vi "Usermgt.vi"(8 "error In":errorcluster) -> (0 "error out":errorcluster)   [LabVIEW 2015]
uses:
  Um- Save.ctl
  Um-Delete.ctl
  Um-Exit.ctl
  <vilib>/addons/database/Connection.llb/DB Tools Open Connec (String).vi
  <vilib>/addons/database/_DB Variant To Data/Database Variant To Data.xnode
  <vilib>/addons/database/NI_Database_API.lvlib
panel:
  in  "Operator ID":string
  out "data":string[](array[string])
  out "User Name 2":string
  out "error out 2":errorcluster
  in  "Exit":T1
  in  "Deleat":T2
  in  "Save":T3
  in  "User Type":string
  in  "User Type":u16(ring) items=["Operator", "Supervisor", "admin"]
  in  "Re-Password":string
  in  "Password":string
  in  "User Name":string
  in  "User Table":i32(listbox)
  # "User Create"
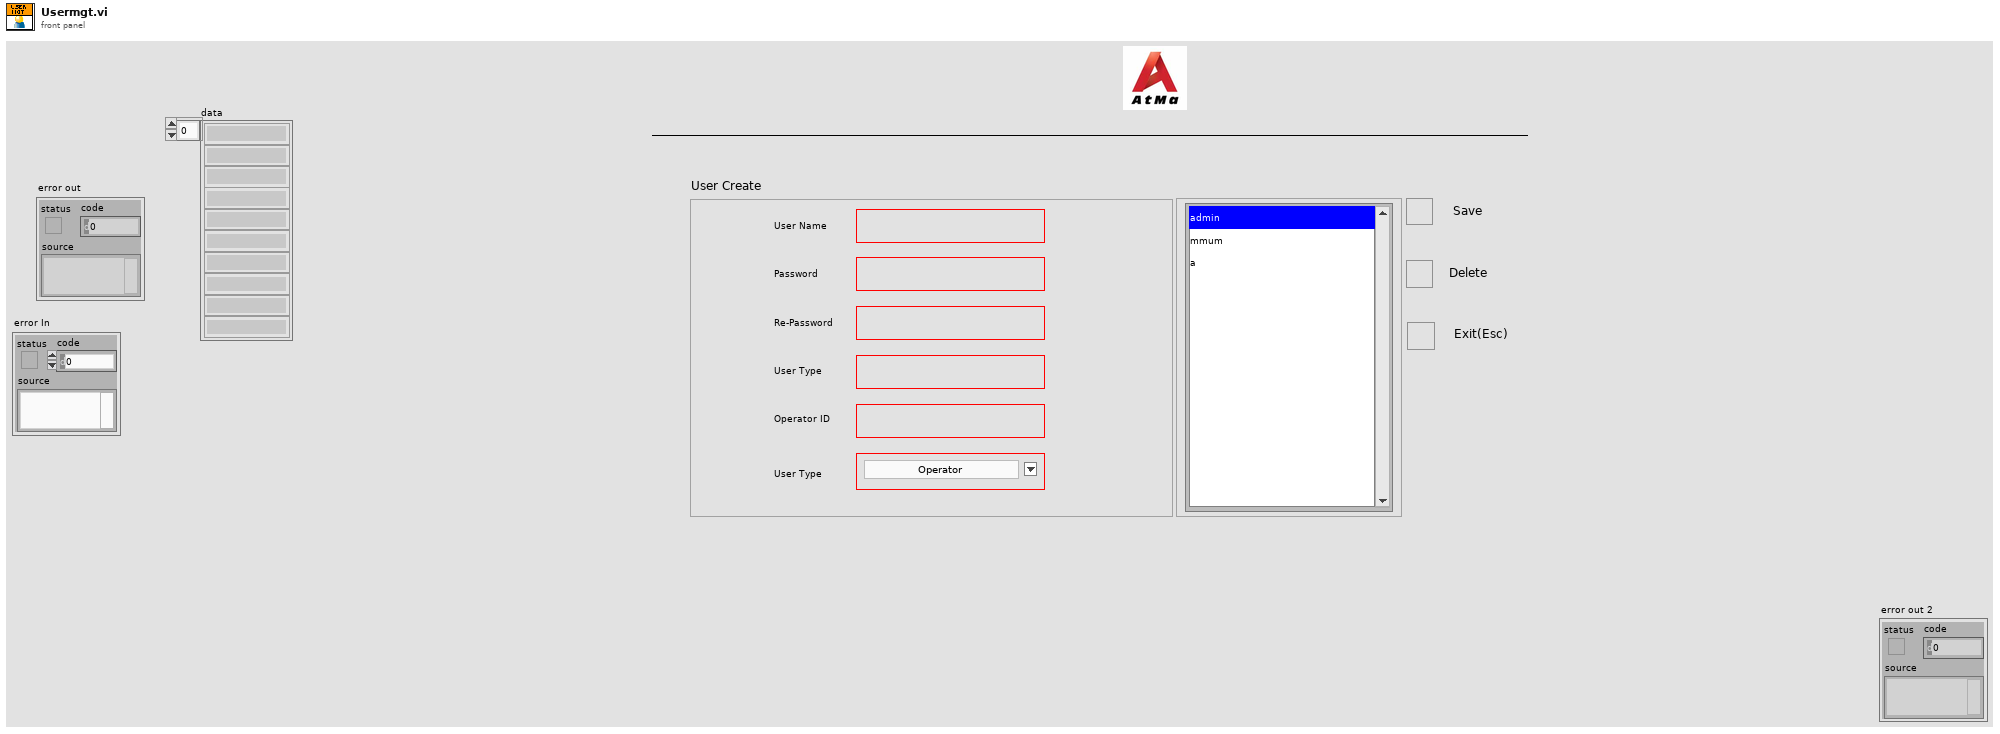
[diagram p1: front panel]
types:
  T1 = typedef "Um-Exit.ctl" = bool
  T2 = typedef "Um-Delete.ctl" = bool
  T3 = typedef "Um- Save.ctl" = bool
  T4 = cluster{"User Name":string, "Password":string, "User Type":string}
  T5 = typedef "NI_Database_API.lvlib/Conn ObjectReference.ctl" = refnum<k1>
  T6 = cluster{"User Name":string, "Password":string, "User Type":string, "Access right":string}
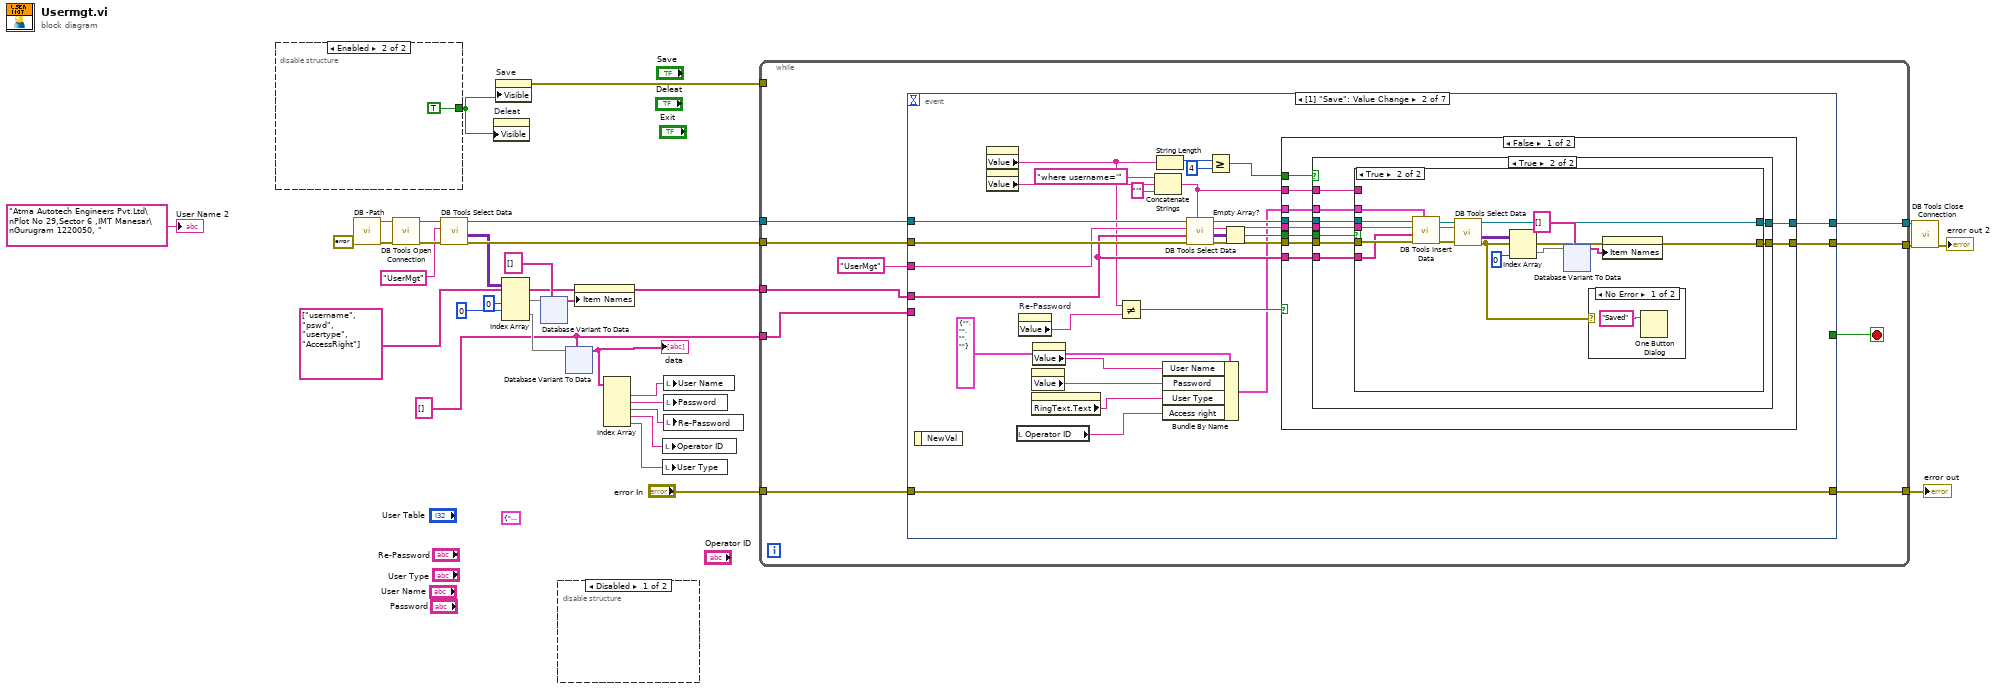
[diagram p0: block diagram]
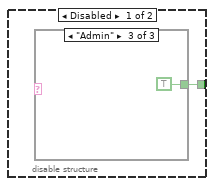
[diagram p3: hidden frame]
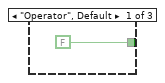
[diagram p4: hidden frame]
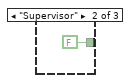
[diagram p5: hidden frame]
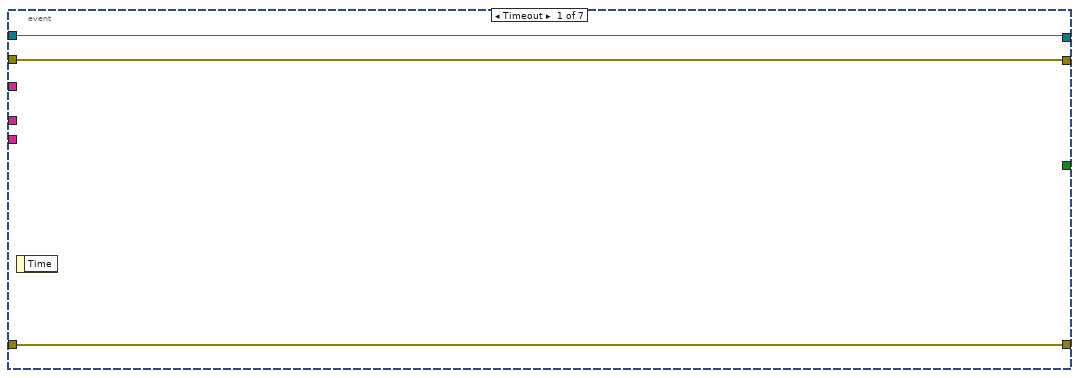
[diagram p6: hidden frame]
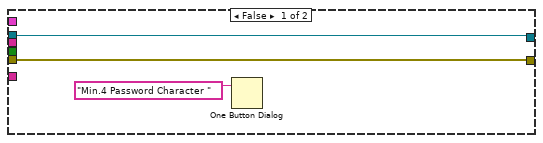
[diagram p7: hidden frame]
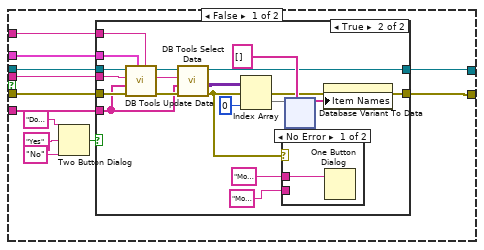
[diagram p8: hidden frame]
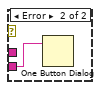
[diagram p10: hidden frame]
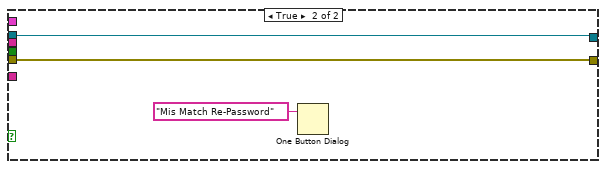
[diagram p12: hidden frame]
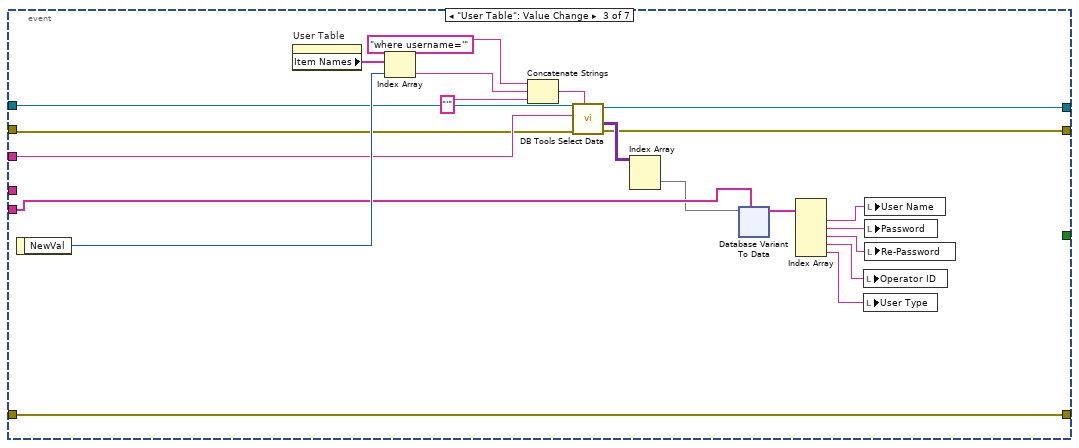
[diagram p13: hidden frame]
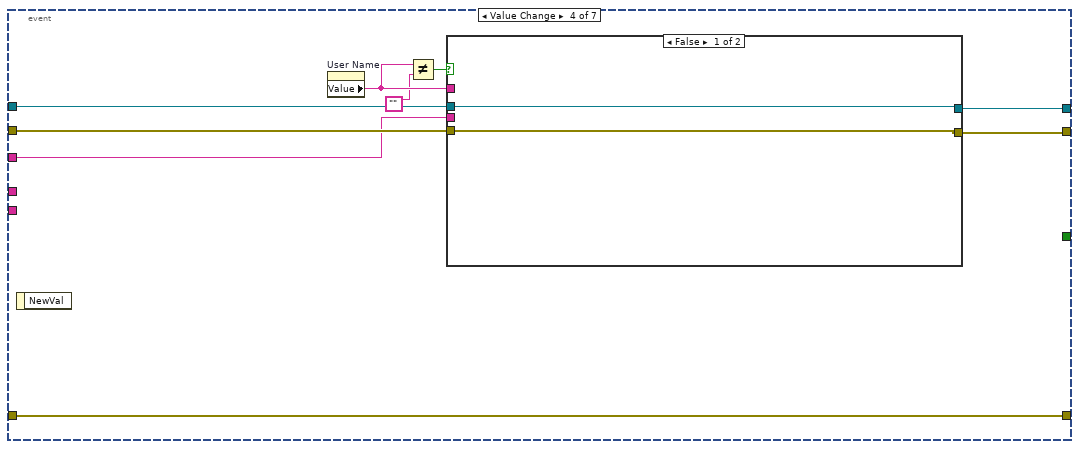
[diagram p14: hidden frame]
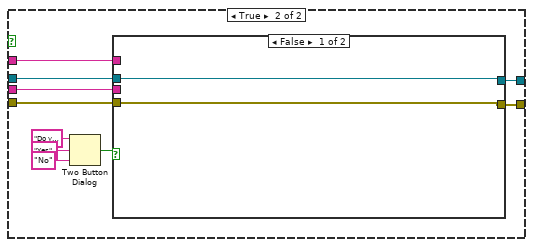
[diagram p15: hidden frame]
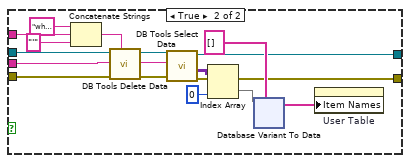
[diagram p16: hidden frame]
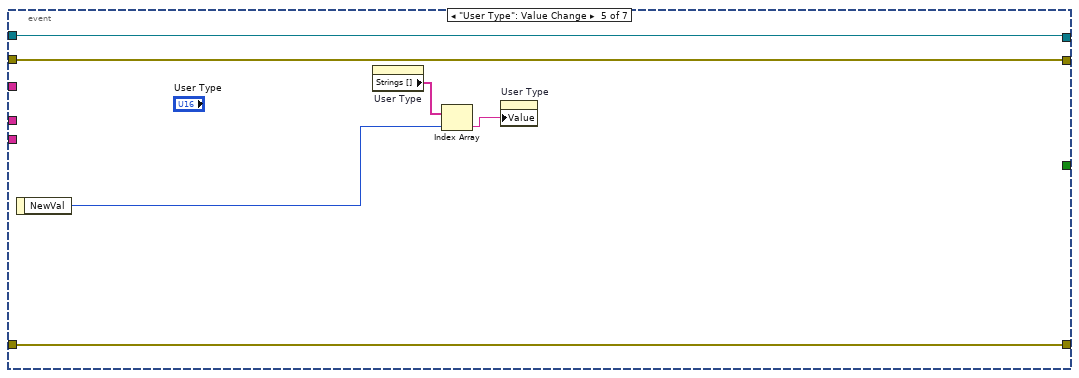
[diagram p17: hidden frame]
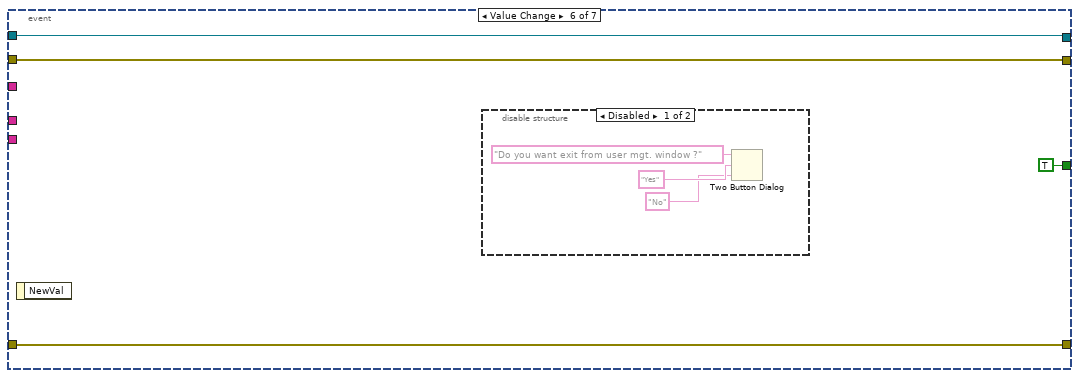
[diagram p18: hidden frame]
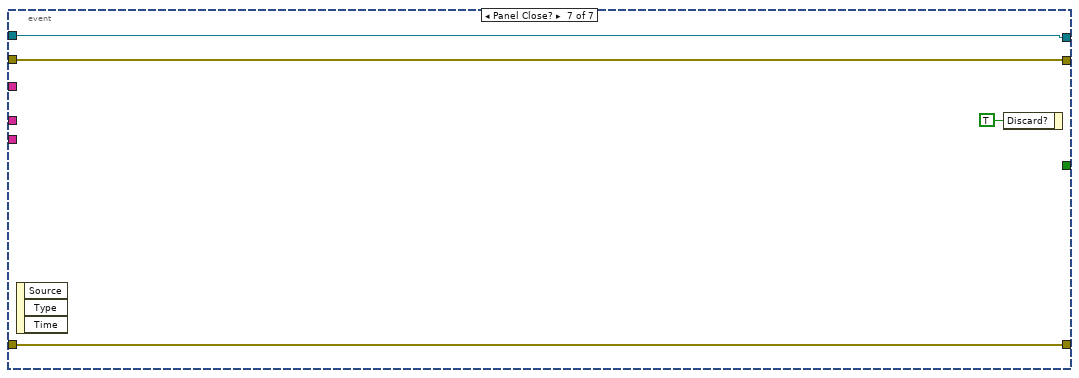
[diagram p20: hidden frame]
diagram:
  w1 = string[] [] ("columns")
  (unwired) T4 {"User Name"="", "Password"="", "User Type"=""} ("Input data")
  n1 = disable-structure shown="Enabled" {
    disable-tunnel: [w31 TRUE] -> w17
    frame Disabled {
      n2 = case shown="\"Admin\"" {
        selector: _ -> [_ _ _]
        tunnel: [FALSE FALSE TRUE] -> w31
        frame "Operator", Default {
        }
        frame "Supervisor" {
        }
        frame "Admin" {
        }
      }
    }
    frame Enabled {
    }
  }
  n3 = call "DB -Path.vi"() -> ("String"=w30:string)  [unwired: 11 in]
  n4 = call-poly <vilib>:"DB Tools Open Connection.vi"("error in (no error)"=errorcluster {"status"=FALSE, "code"=0, "source"=""}, "connection information"=w30) -> ("error out"=w27:errorcluster, "connection reference"=w26:T5)  [unwired: 6 in]
  n5 = call <vilib>:"DB Tools Select Data.vi"("error in (no error)"=w27, "table"="UserMgt", "connection reference"=w26) -> ("error out"=w24:errorcluster, "data"=w18:variant[][], "connection reference out"=w25:T5)  [unwired: 3 in]
  n6 = property on="Deleat" class="Bool (strict)"("Visible"=w17) -> ()  [unwired: 2 in, 2 out]
  n7 = property on="Save" class="Bool (strict)"("Visible"=w17) -> (error out=w16:errorcluster)  [unwired: 2 in, 1 out]
  n8 = Index Array(array=w18, index (col) #1=0 ("disabled index (col)"), index (row) #2=0 ("disabled index (row)")) -> (element #1=w22:variant[], element #2=w8:variant[])  [unwired: 2 in]
  n9 = xnode "Database Variant To Data"("database variant"=w22, "type"=string[] []) -> ("data"=w19:string[])  [unwired: 1 in, 1 out]
  n10 = disable-structure shown="Disabled" {
    frame Disabled {
    }
    frame Enabled {
    }
  }
  n11 = xnode "Database Variant To Data"("database variant"=w8, "type"=w1) -> ("data"=w7:string[])  [unwired: 1 in, 1 out]
  "data" <- w7
  n12 = property on="User Table" class="LstBox (strict)"("Item Names"=w19) -> ()  [unwired: 2 in, 2 out]
  n13 = Index Array(array=w7) -> (element #1=w6:string, element #2=w5:string, element #3=w4:string, element #4=w2:string, element #5=w3:string)  [unwired: 5 in]
  n14 = local write "Operator ID"(w2) -> ()
  n15 = local write "User Type"(w3) -> ()
  n16 = local write "User Name"(w6) -> ()
  n17 = local write "Password"(w5) -> ()
  n18 = local write "Re-Password"(w4) -> ()
  n19 = while {
    tunnel: w25 -> [w44]
    tunnel: w24 -> [w43]
    tunnel: [w41] -> w29
    tunnel: [w40] -> w28
    tunnel: w16 -> [_]
    tunnel: string[] ["username", "pswd", "usertype", "AccessRight"] ("columns") -> [w39]
    tunnel: "error In" -> [w38]
    tunnel: [w37] -> w12
    tunnel: w1 -> [w36]
    stop <- w45 stop-if-true
    n20 = event shown="[1] \"Save\": Value Change" {
      selector: _ -> [_ _ _ _ _ _ _]
      dyn-events: _ -> [_ _ _ _ _ _ _]
      timeout: _ -> [_ _ _ _ _ _ _]
      tunnel: [_ _ _ _ _ TRUE ("T button?") _] -> w45
      tunnel: w44 -> [w48 w75 w237 w292 w363 w370 w375]
      tunnel: w43 -> [w47 w74 w236 w291 w362 w369 w374]
      tunnel: "UserMgt" ("table") -> [_ w67 w239 w287 _ _ _]
      tunnel: w39 -> [_ w66 _ _ _ _ _]
      tunnel: [w48 w65 w235 w285 w363 w370 w375] -> w41
      tunnel: [w47 w64 w234 w284 w362 w369 w374] -> w40
      tunnel: w38 -> [w46 w50 w233 w286 w361 w367 w376]
      tunnel: [w46 w50 w233 w286 w361 w367 w376] -> w37
      tunnel: w36 -> [_ _ w227 _ _ _ _]
      event Timeout {
        n21 = event-data() -> ()  [unwired: 1 in, 1 out]
      }
      event Value Change {
        n22 = event-data() -> ()  [unwired: 1 in, 1 out]
        n23 = property on="Password" class="Str"() -> ("Value"=w52:string)  [unwired: 2 in, 2 out]
        n24 = property on="User Name" class="Str"() -> ("Value"=w51:string)  [unwired: 2 in, 2 out]
        n25 = local read "Operator ID"() -> (w49:string)
        n26 = property on="Re-Password" class="Str"() -> ("Value"=w58:string)  [unwired: 2 in, 2 out]
        n27 = property on="User Type" class="Ring (strict)"() -> ("RingText.Text"=w55:string)  [unwired: 2 in, 2 out]
        n28 = property on="Password" class="Str"() -> ("Value"=w57:string)  [unwired: 2 in, 2 out]
        n29 = property on="User Name" class="Str"() -> ("Value"=w56:string)  [unwired: 2 in, 2 out]
        n30 = Not Equal?(x=w52, y=w58) -> (x != y?=w59:bool)
        n31 = Concatenate Strings("where username='" ("condition"), w51, "'" ("User Name")) -> (w63:string)
        n32 = String Length(string=w52) -> (length=w62:i32)
        n33 = Bundle By Name(cluster=T6 {"User Name"="", "Password"="", "User Type"="", "Access right"=""} ("input cluster"), "User Name"=w56, "Password"=w57, "User Type"=w55, "Access right"=w49) -> (w53:T6)
        n34 = call <vilib>:"DB Tools Select Data.vi"("condition"=w63, "error in (no error)"=w74, "columns"=w66, "table"=w67, "connection reference"=w75) -> ("error out"=w68:errorcluster, "data"=w73:variant[][], "connection reference out"=w69:T5)  [unwired: 1 in]
        n35 = Greater Or Equal?(x=w62, y=4) -> (x >= y?=w60:bool)
        n36 = Empty Array?(array=w73) -> (empty?=w72:bool)
        n37 = case shown="False" w59 {
          tunnel: w72 -> [w85 _]
          tunnel: w69 -> [w84 w224]
          tunnel: w68 -> [w83 w223]
          tunnel: w67 -> [w82 _]
          tunnel: w66 -> [w81 _]
          tunnel: w53 -> [w80 _]
          tunnel: [w79 w224] -> w65
          tunnel: [w78 w223] -> w64
          tunnel: w63 -> [w77 _]
          tunnel: w60 -> [w76 _]
          frame False {
            n38 = case shown="True" w76 {
              tunnel: w85 -> [_ w97]
              tunnel: w84 -> [w88 w96]
              tunnel: w83 -> [w87 w95]
              tunnel: w82 -> [_ w94]
              tunnel: w81 -> [_ w93]
              tunnel: w80 -> [_ w92]
              tunnel: [w88 w91] -> w79
              tunnel: [w87 w90] -> w78
              tunnel: w77 -> [_ w89]
              frame False {
                n39 = One Button Dialog(message="Min.4 Password Character ") -> ()  [unwired: 1 in, 1 out]
              }
              frame True {
                n40 = case shown="True" w97 {
                  tunnel: w96 -> [w109 w182]
                  tunnel: w95 -> [w108 w181]
                  tunnel: w94 -> [w103 w176]
                  tunnel: w93 -> [w100 w180]
                  tunnel: w92 -> [w101 w179]
                  tunnel: [w99 w170] -> w91
                  tunnel: [w98 w169] -> w90
                  tunnel: w89 -> [w102 _]
                  frame False {
                    n41 = Two Button Dialog(message="Do you want  modification" ("T button name (\"OK\")"), 1:"No" ("F button name (\"Cancel\")"), 2:"Yes" ("T button name (\"OK\")")) -> (T button?=w107:bool)
                    n42 = case shown="True" w107 {
                      tunnel: w109 -> [w111 w128]
                      tunnel: w108 -> [w110 w127]
                      tunnel: w103 -> [_ w122]
                      tunnel: w102 -> [_ w126]
                      tunnel: w101 -> [_ w125]
                      tunnel: w100 -> [_ w116]
                      tunnel: [w111 w115] -> w99
                      tunnel: [w110 w114] -> w98
                      frame False {
                      }
                      frame True {
                        n43 = call <vilib>:"DB Tools Update Data.vi"("condition"=w126, "data"=w125, "error in (no error)"=w127, "columns"=w116, "table"=w122, "connection reference"=w128) -> ("error out"=w123:errorcluster, "connection reference out"=w124:T5)  [unwired: 4 in]
                        n44 = call <vilib>:"DB Tools Select Data.vi"("error in (no error)"=w123, "columns"=w116, "table"=w122, "connection reference"=w124) -> ("error out"=w114:errorcluster, "data"=w121:variant[][], "connection reference out"=w115:T5)  [unwired: 2 in]
                        n45 = Index Array(array=w121, index (col)=0 ("disabled index (col)")) -> (element=w119:variant[])  [unwired: 1 in]
                        n46 = case shown="No Error" w114 {
                          tunnel: "Modification is Successfully" ("T button name (\"OK\")") -> [w129 _]
                          tunnel: "Modification is Unsuccessfully" ("T button name (\"OK\")") -> [_ w130]
                          frame No Error {
                            n47 = One Button Dialog(message=w129) -> ()  [unwired: 1 in, 1 out]
                          }
                          frame Error {
                            n48 = One Button Dialog(message=w130) -> ()  [unwired: 1 in, 1 out]
                          }
                        }
                        n49 = xnode "Database Variant To Data"("database variant"=w119, "type"=string[] []) -> ("data"=w117:string[])  [unwired: 1 in, 1 out]
                        n50 = property on="User Table" class="LstBox (strict)"("Item Names"=w117) -> ()  [unwired: 2 in, 2 out]
                      }
                    }
                  }
                  frame True {
                    n51 = call <vilib>:"DB Tools Insert Data.vi"("data"=w179, "error in (no error)"=w181, "columns"=w180, "table"=w176, "connection reference"=w182) -> ("error out"=w177:errorcluster, "connection reference out"=w178:T5)  [unwired: 5 in]
                    n52 = call <vilib>:"DB Tools Select Data.vi"("error in (no error)"=w177, "table"=w176, "connection reference"=w178) -> ("error out"=w169:errorcluster, "data"=w175:variant[][], "connection reference out"=w170:T5)  [unwired: 3 in]
                    n53 = Index Array(array=w175, index (col)=0 ("disabled index (col)")) -> (element=w173:variant[])  [unwired: 1 in]
                    n54 = xnode "Database Variant To Data"("database variant"=w173, "type"=string[] []) -> ("data"=w171:string[])  [unwired: 1 in, 1 out]
                    n55 = case shown="No Error" w169 {
                      frame No Error {
                        n56 = One Button Dialog(message="Saved" ("T button name (\"OK\")")) -> ()  [unwired: 1 in, 1 out]
                      }
                      frame Error {
                      }
                    }
                    n57 = property on="User Table" class="LstBox (strict)"("Item Names"=w171) -> ()  [unwired: 2 in, 2 out]
                  }
                }
              }
            }
          }
          frame True {
            n58 = One Button Dialog(message="Mis Match Re-Password") -> ()  [unwired: 1 in, 1 out]
          }
        }
      }
      event "User Table": Value Change {
        n59 = event-data() -> ("NewVal"=w243:i32)  [unwired: 1 in]
        n60 = property on="User Table" class="LstBox (strict)"() -> ("Item Names"=w244:string[])  [unwired: 2 in, 2 out]
        n61 = Index Array(array=w244, index=w243) -> (element=w241:string)
        n62 = Concatenate Strings("where username='" ("condition"), w241, "'" ("User Name")) -> (w240:string)
        n63 = call <vilib>:"DB Tools Select Data.vi"("condition"=w240, "error in (no error)"=w236, "table"=w239, "connection reference"=w237) -> ("error out"=w234:errorcluster, "data"=w238:variant[][], "connection reference out"=w235:T5)  [unwired: 2 in]
        n64 = Index Array(array=w238) -> (element=w226:variant[])  [unwired: 2 in]
        n65 = xnode "Database Variant To Data"("database variant"=w226, "type"=w227) -> ("data"=w225:string[])  [unwired: 1 in, 1 out]
        n66 = Index Array(array=w225) -> (element #1=w228:string, element #2=w229:string, element #3=w230:string, element #4=w232:string, element #5=w231:string)  [unwired: 5 in]
        n67 = local write "Operator ID"(w232) -> ()
        n68 = local write "User Type"(w231) -> ()
        n69 = local write "User Name"(w228) -> ()
        n70 = local write "Password"(w229) -> ()
        n71 = local write "Re-Password"(w230) -> ()
      }
      event Value Change {
        n72 = event-data() -> ()  [unwired: 1 in, 1 out]
        n73 = property on="User Name" class="Str"() -> ("Value"=w290:string)  [unwired: 2 in, 2 out]
        n74 = Not Equal?(x=w290, y="") -> (x != y?=w288:bool)
        n75 = case shown="False" w288 {
          tunnel: w292 -> [w294 w300]
          tunnel: w291 -> [w293 w299]
          tunnel: w290 -> [_ w298]
          tunnel: w287 -> [_ w297]
          tunnel: [w294 w296] -> w285
          tunnel: [w293 w295] -> w284
          frame False {
          }
          frame True {
            n76 = Two Button Dialog(message="Do you want delete the user id & password", 1:"No" ("F button name (\"Cancel\")"), 2:"Yes" ("T button name (\"OK\")")) -> (T button?=w301:bool)
            n77 = case shown="False" w301 {
              tunnel: w300 -> [w306 w322]
              tunnel: w299 -> [w305 w321]
              tunnel: w298 -> [_ w317]
              tunnel: w297 -> [_ w314]
              tunnel: [w306 w308] -> w296
              tunnel: [w305 w307] -> w295
              frame False {
              }
              frame True {
                n78 = Concatenate Strings("where username='" ("condition"), w317, "'" ("User Name")) -> (w318:string)
                n79 = call <vilib>:"DB Tools Delete Data.vi"("condition"=w318, "error in (no error)"=w321, "table"=w314, "connection reference"=w322) -> ("error out"=w315:errorcluster, "connection reference out"=w316:T5)  [unwired: 6 in]
                n80 = call <vilib>:"DB Tools Select Data.vi"("error in (no error)"=w315, "table"=w314, "connection reference"=w316) -> ("error out"=w307:errorcluster, "data"=w312:variant[][], "connection reference out"=w308:T5)  [unwired: 3 in]
                n81 = Index Array(array=w312, index (col)=0 ("disabled index (col)")) -> (element=w311:variant[])  [unwired: 1 in]
                n82 = xnode "Database Variant To Data"("database variant"=w311, "type"=string[] []) -> ("data"=w309:string[])  [unwired: 1 in, 1 out]
                n83 = property on="User Table" class="LstBox (strict)"("Item Names"=w309) -> ()  [unwired: 2 in, 2 out]
              }
            }
          }
        }
      }
      event "User Type": Value Change {
        n84 = event-data() -> ("NewVal"=w366:u16)  [unwired: 1 in]
        n85 = property on="User Type" class="Ring (strict)"() -> ("Strings []"=w365:string[])  [unwired: 2 in, 2 out]
        n86 = Index Array(array=w365, index=w366) -> (element=w364:string)
        n87 = property on="User Type" class="Str"("Value"=w364) -> ()  [unwired: 2 in, 2 out]
      }
      event Value Change {
        n88 = event-data() -> ()  [unwired: 1 in, 1 out]
        n89 = disable-structure shown="Disabled" {
          frame Disabled {
            n90 = Two Button Dialog(message="Do you want exit from user mgt. window ?", 1:"No" ("F button name (\"Cancel\")"), 2:"Yes" ("T button name (\"OK\")")) -> ()  [unwired: 1 out]
          }
          frame Enabled {
          }
        }
      }
      event Panel Close? {
        n91 = event-data() -> ()  [unwired: 1 in, 3 out]
        n92 = event-data("Discard?"=TRUE) -> ()  [unwired: 1 in, 1 out]
      }
    }
  }
  "error out" <- w12
  n93 = call <vilib>:"DB Tools Close Connection.vi"("error in (no error)"=w28, "connection reference"=w29) -> ("error out"=→"error out 2":errorcluster)  [unwired: 5 in]
  "User Name 2" <- "Atma Autotech Engineers Pvt.Ltd\nPlot No 29,Sector 6 ,IMT Manesar\nGurugram 1220050, " ("string")
